vi "SearchAndReplaceEx.vi"(4 "Options":u32 format="%.0x", 5 "replace all? (F)":bool, 6 "offset":i32, 7 "substring to replace":i32, 8 "error in":errorcluster, 9 "replace string":string, 10 "search pattern":string, 11 "string":string) -> (0 "error out":errorcluster, 1 "offset past replacement":i32, 2 "number of replacements":i32, 3 "string":string)   [LabVIEW 2021, in "libpcre2-8.lvlib"]
uses:
  libpcre2-8.lvlib
  Pcre2GetOvectorPointer8.vi
  Pcre2MoOfSubstrNumFmOv.vi
  Pcre2SubstringFromSubjectByOffsets (s).vi
  Pcre2JitCompile8.vi
  Pcre2JitMatch8.vi
  Pcre2CompileError.vi
  Pcre2FnkCallError.vi
  Pcre2ErrorNull.vi
  Pcre2LibError.vi
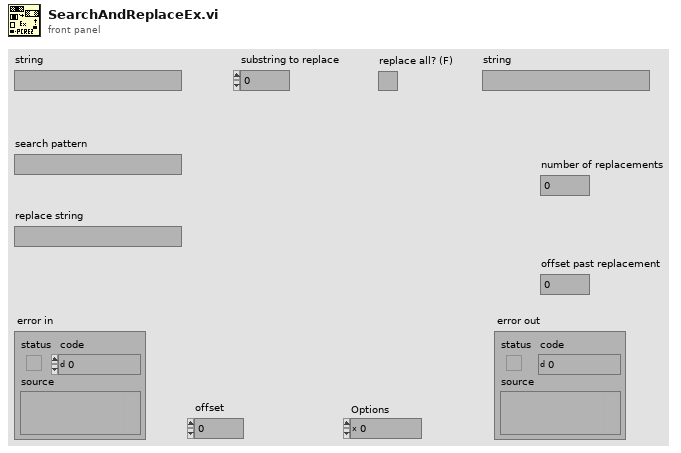
[diagram p1: front panel]
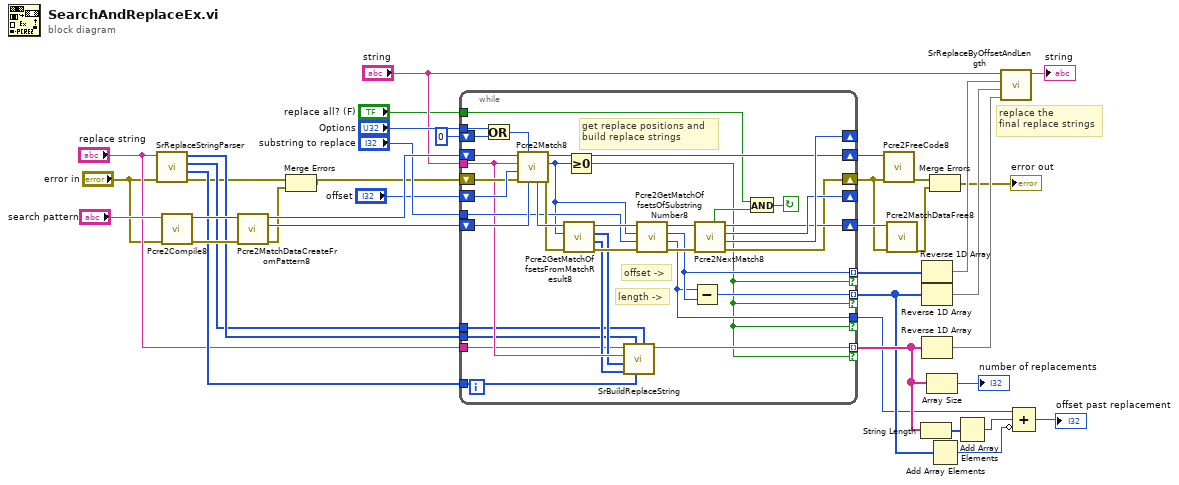
[diagram p0: block diagram]
diagram:
  # "replace the \nfinal replace strings"
  n1 = call "SrReplaceStringParser.vi"("error in"="error in", "ReplaceString"="replace string") -> ("error out"=w3:errorcluster, "ReplSubStrNum"=w10:i32[], "ReplStrLengths"=w11:i32[], "ReplStrOffsets"=w12:i32[])  [unwired: 6 in]
  n2 = call "Pcre2Compile8.vi"("error in"="error in", "Pattern"="search pattern") -> ("error out"=w13:errorcluster, "pCode"=w14:u64)  [unwired: 8 in]
  n3 = call "Pcre2MatchDataCreateFromPattern8.vi"("error in"=w13, "pCode"=w14) -> ("error out"=w2:errorcluster, "pMatchData"=w38:u64, "pCode"=w37:u64)  [unwired: 7 in]
  n4 = Merge Errors(w3, w2) -> (w4:errorcluster)
  n5 = while {
    tunnel: "string" -> [w46]
    shift-right: [w69] -> _
    shift-left: "offset" -> [w72]
    shift-right: [w67] -> w32
    shift-left: w38 -> [w71]
    shift-right: [w70] -> _
    shift-left: u32 0 ("GlobalOptions") -> [w54]
    shift-right: [w68] -> w33
    shift-left: w37 -> [w73]
    shift-right: [w65] -> w31
    shift-left: w4 -> [w66]
    tunnel: "replace string" -> [w43]
    tunnel: w10 -> [w40]
    tunnel: w12 -> [w42]
    tunnel: w11 -> [w41]
    tunnel: "substring to replace" -> [w61]
    tunnel: [w47] -> w22 mode=indexing if=w39
    tunnel: [w57] -> w21 mode=indexing if=w39
    tunnel: [w56] -> w35 mode=indexing if=w39
    tunnel: "Options" -> [w52]
    tunnel: [w51] -> w19 if=w39
    tunnel: "replace all? (F)" -> [w50]
    stop <- w48 continue-if-true
    # "get replace positions and \nbuild replace strings"
    # "length ->"
    # "offset ->"
    n6 = Or(x=w52, y=w54) -> (x .or. y?=w53:u32)
    n7 = call "Pcre2Match8.vi"("pMatchData"=w71, "Options"=w53, "error in"=w66, "StartOffset"=w72, "Subject"=w46, "pCode"=w73) -> ("error out"=w63:errorcluster, "MatchResult"=w58:i32, "pCode"=w68:u64, "pMatchData"=w64:u64)  [unwired: 2 in]
    n8 = call "Pcre2GetMatchOffsetsFromMatchResult8.vi"("error in"=w63, "MatchResult"=w58, "pMatchData"=w64) -> ("error out"=w55:errorcluster, "OffsetsPastMatch"=w44:i32[], "MatchOffsets"=w45:i32[], "pMatchData"=w62:u64)  [unwired: 5 in]
    n9 = Greater Or Equal To 0?(x=w58) -> (x >= 0?=w39:bool)
    n10 = call "SrBuildReplaceString.vi"("ReplStrLengths"=w41, "ReplSubStrNum"=w40, "ReplStrOffsets"=w42, "OffsetsPastMatch"=w44, "MatchOffsets"=w45, "Subject"=w46, "ReplaceString"=w43) -> ("ReplaceString"=w47:string)  [unwired: 4 in]
    n11 = call "Pcre2GetMatchOffsetsOfSubstringNumber8.vi"("error in"=w55, "Number"=w61, "MatchResult"=w58, "pMatchData"=w62) -> ("error out"=w59:errorcluster, "OffsetPastMatch"=w51:i32, "MatchOffset"=w56:i32, "pMatchData"=w60:u64)  [unwired: 4 in]
    n12 = Subtract(x=w51, y=w56) -> (x-y=w57:i32)
    n13 = call "Pcre2NextMatch8.vi"("error in"=w59, "pMatchData"=w60) -> ("error out"=w65:errorcluster, "GlobalOptions"=w70:u32, "NextStartOffset"=w69:u64, "pMatchData"=w67:u64, "ContinueMatch?"=w49:bool)  [unwired: 5 in]
    n14 = And(x=w50, y=w49) -> (x .and. y?=w48:bool)
  }
  n15 = call "Pcre2FreeCode8.vi"("error in"=w31, "pCode"=w33) -> ("error out"=w30:errorcluster)  [unwired: 9 in]
  n16 = call "Pcre2MatchDataFree8.vi"("error in"=w31, "pMatchData"=w32) -> ("error out"=w29:errorcluster)  [unwired: 9 in]
  n17 = String Length(string=w22) -> (length=w20:i32[])
  n18 = Reverse 1D Array(array=w35) -> (reversed array=w7:i32[])
  n19 = Reverse 1D Array(array=w21) -> (reversed array=w34:i32[])
  n20 = Reverse 1D Array(array=w22) -> (reversed array=w6:string[])
  n21 = Array Size(array=w22) -> (size(s)=→"number of replacements":i32)
  n22 = Merge Errors(w30, w29) -> (→"error out":errorcluster)
  n23 = Add Array Elements(numeric array=w21) -> (sum=w18:i32)
  n24 = Add Array Elements(numeric array=w20) -> (sum=w16:i32)
  n25 = call "SrReplaceByOffsetAndLength.vi"("Replace"=w6, "Lengths"=w34, "Offsets"=w7, "String"="string") -> ("String"=→"string":string)  [unwired: 7 in]
  n26 = Compound Arithmetic op=ADD(w19, w16, invert w18) -> (→"offset past replacement":i32)
